vi "AB_RW_Project_InteropAssembly_Info.vi"(7 "action":T3, 8 "error in (no error)":errorcluster, 10 "InteropAssebly info in":T2, 11 "Object In":T1) -> (0 "error out":errorcluster, 2 "InteropAssebly info out":T2, 3 "Object Out":T1)   [LabVIEW 2020]
uses:
  <vilib>/AppBuilder/RW_Project/AB_RW_Project_PropBag_Action.ctl
  <vilib>/AppBuilder/RW_Project/AB_RW_Project_InteropAssembly_Data.ctl
  <resource>/Framework/Providers/API/ItemRef.ctl
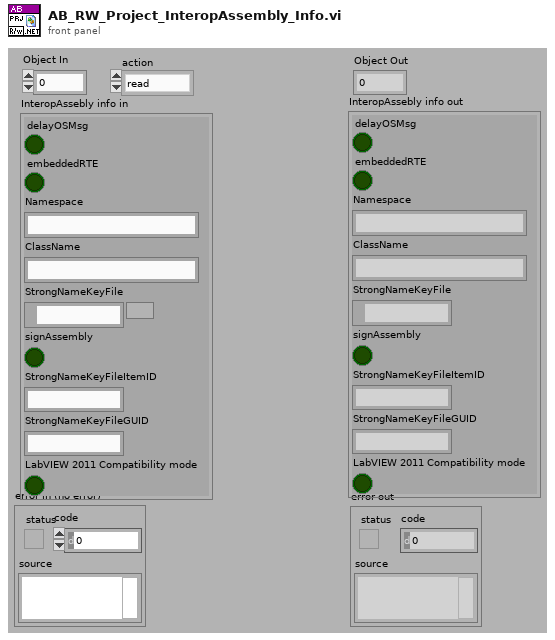
[diagram p1: front panel]
types:
  T1 = typedef "ItemRef.ctl" = u64
  T2 = typedef "AB_RW_Project_InteropAssembly_Data.ctl" = cluster{"delayOSMsg":bool, "embeddedRTE":bool, "Namespace":string, "ClassName":string, "StrongNameKeyFile":path, "signAssembly":bool, "StrongNameKeyFileItemID":string, "StrongNameKeyFileGUID":string, "LabVIEW 2011 Compatibility mode":bool}
  T3 = typedef "AB_RW_Project_PropBag_Action.ctl" = enum16{"read", "write", "clear", "readPrevious", "writePrevious", "clearPrevious"}
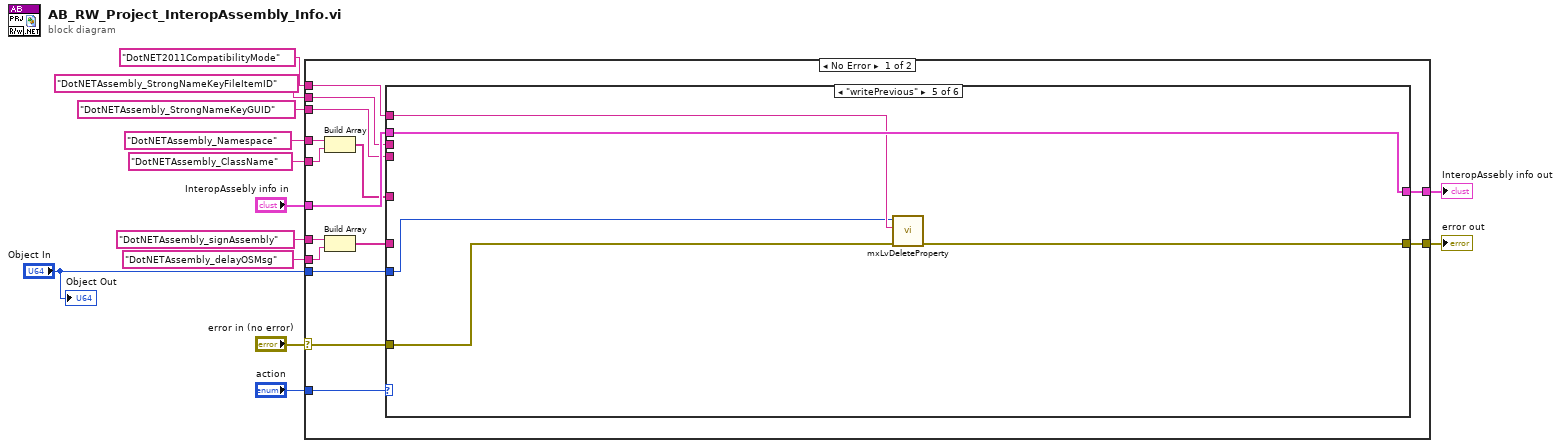
[diagram p0: block diagram]
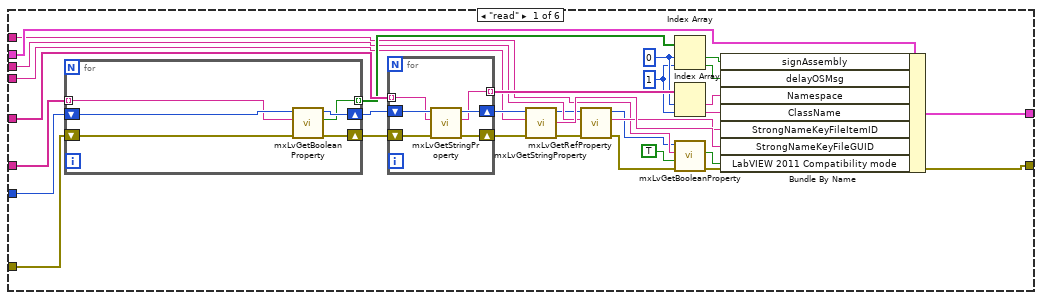
[diagram p2: hidden frame]
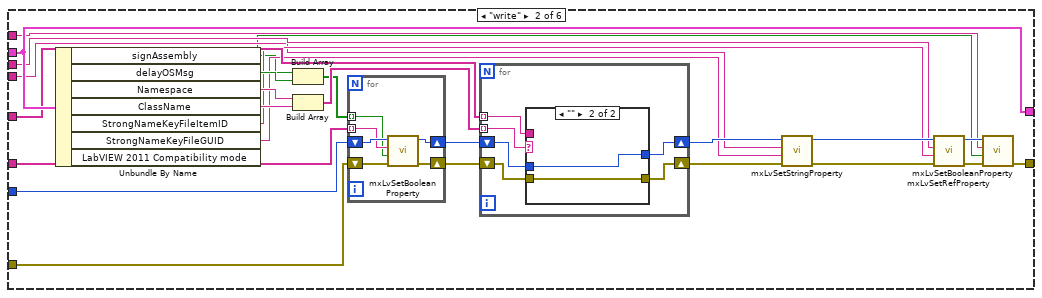
[diagram p3: hidden frame]
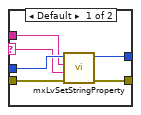
[diagram p4: hidden frame]
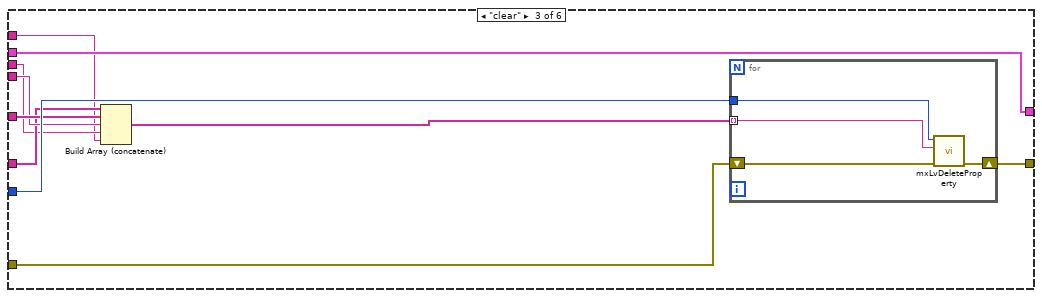
[diagram p5: hidden frame]
diagram:
  n1 = case shown="No Error" "error in (no error)" {
    selector: "error in (no error)" -> [w18 w141]
    tunnel: "Object In" -> [w27 _]
    tunnel: [w28 w140] -> w8
    tunnel: "InteropAssebly info in" -> [w26 w140]
    tunnel: "action" -> [w25 _]
    tunnel: "DotNETAssembly_Namespace" -> [w24 _]
    tunnel: "DotNETAssembly_ClassName" -> [w23 _]
    tunnel: "DotNETAssembly_StrongNameKeyGUID" -> [w21 _]
    tunnel: "DotNETAssembly_delayOSMsg" -> [w20 _]
    tunnel: [w17 w141] -> w4
    tunnel: "DotNETAssembly_StrongNameKeyFileItemID" -> [w16 _]
    tunnel: "DotNETAssembly_signAssembly" -> [w15 _]
    tunnel: "DotNET2011CompatibilityMode" -> [w14 _]
    frame No Error {
      n2 = Build Array(w24, w23) -> (w22:string[])
      n3 = Build Array(w15, w20) -> (w19:string[])
      n4 = case shown="\"writePrevious\"" w25 {
        tunnel: [w55 w93 w126 w132 w137 w139] -> w28
        tunnel: w27 -> [w52 w92 w125 _ w133 _]
        tunnel: w26 -> [w56 w93 w126 w132 w137 w139]
        tunnel: w22 -> [w57 w87 w123 _ _ _]
        tunnel: w21 -> [w44 w78 w122 _ _ _]
        tunnel: w19 -> [w50 w91 w121 _ _ _]
        tunnel: w18 -> [w48 w86 w120 w131 w135 w138]
        tunnel: [w33 w74 w119 w131 w134 w138] -> w17
        tunnel: w16 -> [w41 w79 w118 _ _ _]
        tunnel: w14 -> [w30 w72 w117 _ w136 _]
        frame "read" {
          w36 = 1 ("index")
          w46 = 0 ("index")
          n5 = for {
            shift-right: [w63] -> w51
            shift-left: w52 -> [w64]
            tunnel: w50 -> [w62] mode=indexing
            tunnel: [w61] -> w49 mode=indexing
            shift-right: [w59] -> w47
            shift-left: w48 -> [w60]
            n6 = call <resource>:"mxLvGetBooleanProperty.vi"("error in"=w60, "Tag"=w62, "Item"=w64) -> ("error out"=w59:errorcluster, "Value"=w61:bool, "Item"=w63:T1)  [unwired: 1 in, 5 out]
          }
          n7 = for {
            shift-right: [w69] -> w45
            shift-left: w51 -> [w70]
            tunnel: [w68] -> w58 mode=indexing
            tunnel: w57 -> [w67] mode=indexing
            shift-right: [w65] -> w43
            shift-left: w47 -> [w66]
            n8 = call <resource>:"mxLvGetStringProperty.vi"("Error In"=w66, "Tag"=w67, "Item"=w70) -> ("Error Out"=w65:errorcluster, "Value"=w68:string, "Item"=w69:T1)  [unwired: 6 out]
          }
          n9 = call <resource>:"mxLvGetStringProperty.vi"("Error In"=w43, "Tag"=w44, "Item"=w45) -> ("Error Out"=w39:errorcluster, "Value"=w42:string, "Item"=w38:T1)  [unwired: 6 out]
          n10 = call <resource>:"mxLvGetRefProperty.vi"("Error In"=w39, "Tag"=w41, "Item"=w38) -> ("Error Out"=w34:errorcluster, "Value"=w40:string, "Item"=w29:T1)  [unwired: 6 out]
          n11 = Index Array(array=w49, index #1=w46, index #2=w36) -> (element #1=w37:bool, element #2=w35:bool)
          n12 = Index Array(array=w58, index #1=w46, index #2=w36) -> (element #1=w54:string, element #2=w53:string)
          n13 = call <resource>:"mxLvGetBooleanProperty.vi"("error in"=w34, "Default Value (F)"=TRUE, "Tag"=w30, "Item"=w29) -> ("error out"=w33:errorcluster, "Value"=w32:bool)  [unwired: 6 out]
          n14 = Bundle By Name(cluster=w56, "signAssembly"=w37, "delayOSMsg"=w35, "Namespace"=w54, "ClassName"=w53, "StrongNameKeyFileItemID"=w40, "StrongNameKeyFileGUID"=w42, "LabVIEW 2011 Compatibility mode"=w32) -> (w55:T2)
        }
        frame "write" {
          n15 = Unbundle By Name(w93) -> ("signAssembly"=w76:bool, "delayOSMsg"=w90:bool, "Namespace"=w96:string, "ClassName"=w95:string, "StrongNameKeyFileItemID"=w80:string, "StrongNameKeyFileGUID"=w77:string, "LabVIEW 2011 Compatibility mode"=w71:bool)
          n16 = Build Array(w76, w90) -> (w89:bool[])
          n17 = Build Array(w96, w95) -> (w94:string[])
          n18 = for {
            shift-right: [w101] -> w88
            shift-left: w92 -> [w102]
            tunnel: w91 -> [w100] mode=indexing
            tunnel: w89 -> [w99] mode=indexing
            shift-right: [w97] -> w85
            shift-left: w86 -> [w98]
            n19 = call <resource>:"mxLvSetBooleanProperty.vi"("error in"=w98, "Value (F)"=w99, "Tag"=w100, "Item"=w102) -> ("error out"=w97:errorcluster, "Item"=w101:T1)  [unwired: 1 in, 5 out]
          }
          n20 = for {
            tunnel: w94 -> [w107] mode=indexing
            shift-right: [w106] -> w84
            shift-left: w88 -> [w108]
            tunnel: w87 -> [w105] mode=indexing
            shift-right: [w103] -> w83
            shift-left: w85 -> [w104]
            n21 = case shown="\"\"" w107 {
              selector: w107 -> [w112 _]
              tunnel: w108 -> [w114 w116]
              tunnel: w105 -> [w111 _]
              tunnel: [w113 w116] -> w106
              tunnel: w104 -> [w110 w115]
              tunnel: [w109 w115] -> w103
              frame Default {
                n22 = call <resource>:"mxLvSetStringProperty.vi"("error in"=w110, "Value (\"\")"=w112, "Tag"=w111, "Item"=w114) -> ("error out"=w109:errorcluster, "Item"=w113:T1)  [unwired: 1 in, 5 out]
              }
              frame "" {
              }
            }
          }
          n23 = call <resource>:"mxLvSetStringProperty.vi"("error in"=w83, "Value (\"\")"=w77, "Tag"=w78, "Item"=w84) -> ("error out"=w82:errorcluster, "Item"=w81:T1)  [unwired: 1 in, 5 out]
          n24 = call <resource>:"mxLvSetRefProperty.vi"("error in"=w82, "Value (\"\")"=w80, "Tag"=w79, "Item"=w81) -> ("error out"=w75:errorcluster, "Item"=w73:T1)  [unwired: 1 in, 5 out]
          n25 = call <resource>:"mxLvSetBooleanProperty.vi"("error in"=w75, "Value (F)"=w71, "Tag"=w72, "Item"=w73) -> ("error out"=w74:errorcluster)  [unwired: 1 in, 6 out]
        }
        frame "clear" {
          n26 = Build Array (concatenate)(w121, w123, w122, w118, w117) -> (w124:string[])
          n27 = for {
            tunnel: w125 -> [w130]
            tunnel: w124 -> [w129] mode=indexing
            shift-right: [w127] -> w119
            shift-left: w120 -> [w128]
            n28 = call <resource>:"mxLvDeleteProperty.vi"("error in"=w128, "Tag"=w129, "Item"=w130) -> ("error out"=w127:errorcluster)  [unwired: 8 out]
          }
        }
        frame "readPrevious" {
        }
        frame "writePrevious" {
          n29 = call <resource>:"mxLvDeleteProperty.vi"("error in"=w135, "Tag"=w136, "Item"=w133) -> ("error out"=w134:errorcluster)  [unwired: 8 out]
        }
        frame "clearPrevious" {
        }
      }
    }
    frame Error {
    }
  }
  "error out" <- w4
  "InteropAssebly info out" <- w8
  "Object Out" <- "Object In"
